vi "Create Polynomial From PFE.vi"(7 "Multiplicity":i32[](array[numeric]), 8 "option":u16(ring)=1 items=["Cancel Co-factors", "Reserve Co-factors"], 9 "Residues":cdb[][](array[numeric]), 10 "Poles":cdb[](array[numeric]), 11 "Polynomial":cdb[](array[numeric])) -> (0 "error":i32, 2 "Denominator":cdb[](array[numeric]), 3 "Numerator":cdb[](array[numeric]))   [LabVIEW 2017, in "NI_AALPro.lvlib"]
doc: "Uses partial fraction expansion to reconstruct a rational polynomial."
uses:
  <vilib>/Analysis/NI_AALPro.lvlib
  <vilib>/Analysis/polynomials.llb/Remove Zero Threshold Type.ctl
  <vilib>/Analysis/polynomials.llb/Add Rational Polynomials (CDB).vi
  <vilib>/Analysis/polynomials.llb/Divide Polynomials (CDB).vi
  <vilib>/Analysis/polynomials.llb/Remove Zero Coefficients (CDB).vi
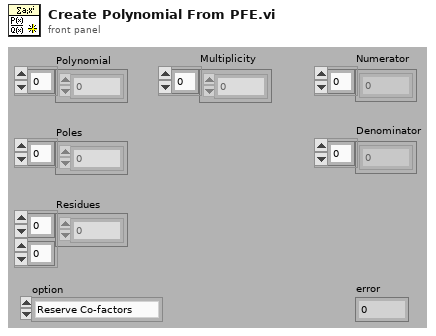
[diagram p1: front panel]
types:
  T1 = typedef "NI_AALPro.lvlib/Remove Zero Threshold Type.ctl" = u16
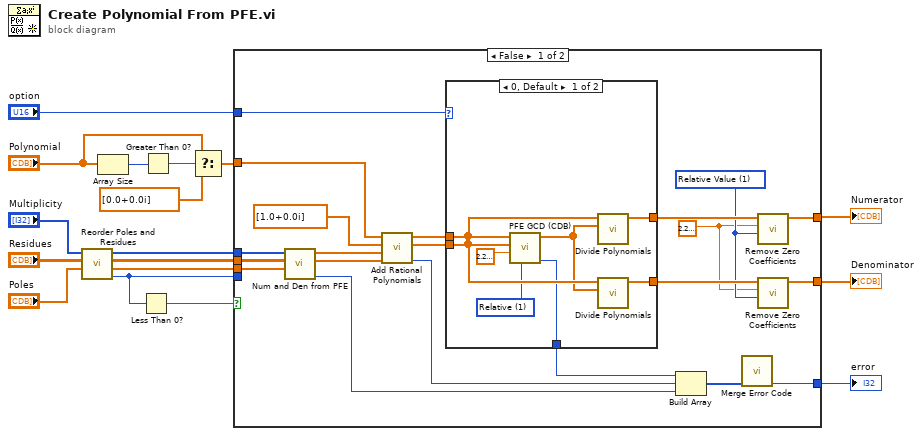
[diagram p0: block diagram]
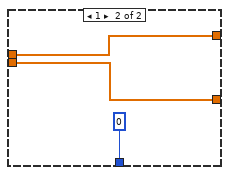
[diagram p2: hidden frame]
diagram:
  n1 = call <vilib>:"Reorder Poles and Residues.vi"("Poles In"="Poles", "Residues In"="Residues", "Multiplicity In"="Multiplicity") -> ("error"=w8:i32, "Poles Out"=w9:cdb[], "Residues Out"=w6:cdb[][], "Multiplicity Out"=w12:i32[])  [unwired: 5 in]
  n2 = Array Size(array="Polynomial") -> (size(s)=w3:i32)
  n3 = Less Than 0?(x=w8) -> (x < 0?=w14:bool)
  n4 = Greater Than 0?(x=w3) -> (x > 0?=w4:bool)
  n5 = Select(t="Polynomial", s=w4, f=cdb[] [0.0+0.0i]) -> (s? t:f=w1:cdb[])
  n6 = case shown="False" w14 {
    tunnel: [w26 w50] -> w17
    tunnel: [w34 _] -> w16
    tunnel: [w33 _] -> w15
    tunnel: w9 -> [w32 _]
    tunnel: w12 -> [w28 _]
    tunnel: w8 -> [_ w50]
    tunnel: "option" -> [w23 _]
    tunnel: w6 -> [w24 _]
    tunnel: w1 -> [w21 _]
    frame False {
      w19 = T1 1 items=["Absolute Value", "Relative Value"] ("threshold type")
      w18 = 2.220446049250313e-16
      n7 = call <vilib>:"Num and Den from PFE.vi"("Poles"=w32, "Residues"=w24, "Multiplicity"=w28) -> ("error"=w25:i32, "Denominator"=w36:cdb[], "Numerator"=w37:cdb[])  [unwired: 6 in]
      n8 = call-poly <vilib>:"Add Rational Polynomials.vi"("Denominator 2"=w36, "Numerator 2"=w37, "Denominator 1"=cdb[] [1.0+0.0i] ("Numerator 1"), "Numerator 1"=w21) -> ("error"=w35:i32, "Denominator Out"=w30:cdb[], "Numerator Out"=w31:cdb[])  [unwired: 5 in]
      n9 = case shown="0, Default" w23 {
        tunnel: [w46 w49] -> w22
        tunnel: [w45 w48] -> w20
        tunnel: w31 -> [w44 w49]
        tunnel: w30 -> [w43 w48]
        tunnel: [w41 0 ("error")] -> w29
        frame 0, Default {
          w42 = u16 1 items=["Absolute", "Relative"] ("tolerance type")
          n10 = call <vilib>:"PFE GCD (CDB).vi"("tolerance type"=w42, "tolerance"=2.220446049250313e-16, "Q(x)"=w43, "P(x)"=w44) -> ("error"=w41:i32, "Greatest Common Divisor"=w40:cdb[])  [unwired: 6 in]
          n11 = call-poly <vilib>:"Divide Polynomials.vi"("Q(x)"=w40, "P(x)"=w44) -> ("P(x)/Q(x)"=w46:cdb[])  [unwired: 7 in, 2 out]
          n12 = call-poly <vilib>:"Divide Polynomials.vi"("Q(x)"=w40, "P(x)"=w43) -> ("P(x)/Q(x)"=w45:cdb[])  [unwired: 7 in, 2 out]
        }
        frame 1 {
        }
      }
      n13 = Build Array(w29, w35, w25) -> (w27:i32[])
      n14 = call <vilib>:"Merge Error Code.vi"("Error Code"=w27) -> ("error code"=w26:i32)  [unwired: 10 in]
      n15 = call-poly <vilib>:"Remove Zero Coefficients.vi"("threshold type"=w19, "threshold"=w18, "P(x) In"=w22) -> ("P(x) Out"=w33:cdb[])  [unwired: 6 in, 2 out]
      n16 = call-poly <vilib>:"Remove Zero Coefficients.vi"("threshold type"=w19, "threshold"=w18, "P(x) In"=w20) -> ("P(x) Out"=w34:cdb[])  [unwired: 6 in, 2 out]
    }
    frame True {
    }
  }
  "Numerator" <- w15
  "Denominator" <- w16
  "error" <- w17
